vi "Move to point.vi"(11 "Point":T2) -> ()   [LabVIEW 2011]
uses:
  point.ctl
  <vilib>/addons/control/pid/pid.llb/PID (DBL).vi
  <vilib>/addons/control/pid/NI_PID_pid.lvlib
panel:
  in  "Y axix PID gains 2":T1={"proportional gain (Kc)"=0.5, "integral time (Ti, min)"=0.1, "derivative time (Td, min)"=0.0}
  in  "X axis PID gains":T1={"proportional gain (Kc)"=2.0, "integral time (Ti, min)"=0.01, "derivative time (Td, min)"=0.0}
  in  "Y scale":dbl
  in  "X scale":dbl
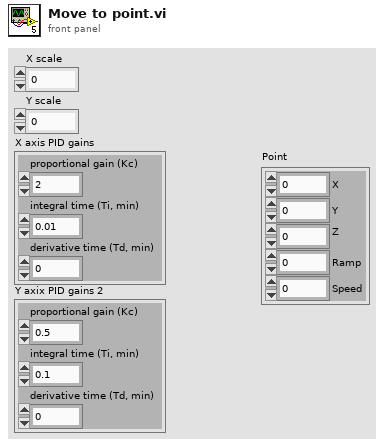
[diagram p1: front panel]
types:
  T1 = cluster{"proportional gain (Kc)":dbl, "integral time (Ti, min)":dbl, "derivative time (Td, min)":dbl}
  T2 = typedef "point.ctl" = cluster{"X":dbl, "Y":dbl, "Z":dbl, "Ramp":dbl, "Speed":dbl}
  T3 = typedef "WPI_EncoderDevRef.ctl" = cluster{"DevStatus":errorcluster, "EncoderIndex":T4, "CounterIndex":T5, "DistancePerCount":dbl, "Decoding Type":T6}
  T4 = typedef "FPGA_EncoderIdx.ctl" = enum8{"Enc 0", "Enc 1", "Enc 2", "Enc 3", "Invalid"}
  T5 = typedef "FPGA_CounterCtrSystemIndex.ctl" = enum8{"Ctr 0", "Ctr 1", "Ctr 2", "Ctr 3", "Ctr 4", "Ctr 5", "Ctr 6", "Ctr 7", "Invalid"}
  T6 = typedef "WPI_EncoderType.ctl" = enum16{"1x", "2x", "4x"}
  T7 = typedef "WPI_MotorControlDeviceRef.ctl" = cluster{"DeviceStatus":errorcluster, "Type":enum16{"PWM", "CAN"}, "PWM":cluster{"Digital Module":T8, "PWM Channel":T9, "DeadBand":T10}, "CAN":cluster{"Device Number":u8, "Control Mode":T11, "Semaphore":T12, "Max Vout":dbl}, "Invert":bool, "TransformRef":T13, "InvTransformRef":T13}
  T8 = typedef "FPGA_TypedefDigitalModule.ctl" = enum16{"Digital Module 1", "Digital Module 2"}
  T9 = typedef "FPGA_DIOPWMChannel.ctl" = enum8{"PWM 1", "PWM 2", "PWM 3", "PWM 4", "PWM 5", "PWM 6", "PWM 7", "PWM 8", "PWM 9", "PWM 10", "Invalid"}
  T10 = typedef "WPI_PWMDeadband.ctl" = cluster{"Name":string, "maxPositivePwm":i32, "minPositivePwm":i32, "centerPwm":i32, "maxNegativePwm":i32, "minNegativePwm":i32, "angularRange":u16}
  T11 = typedef "WPI_CANJaguar_ControlMode.ctl" = enum8{"Percent VBus", "Current", "Speed", "Position", "Voltage"}
  T12 = typedef "Semaphore RefNum" = refnum<k1>
  T13 = typedef "WPI_PWMTransform_ConPane.ctl" = refnum<vi>
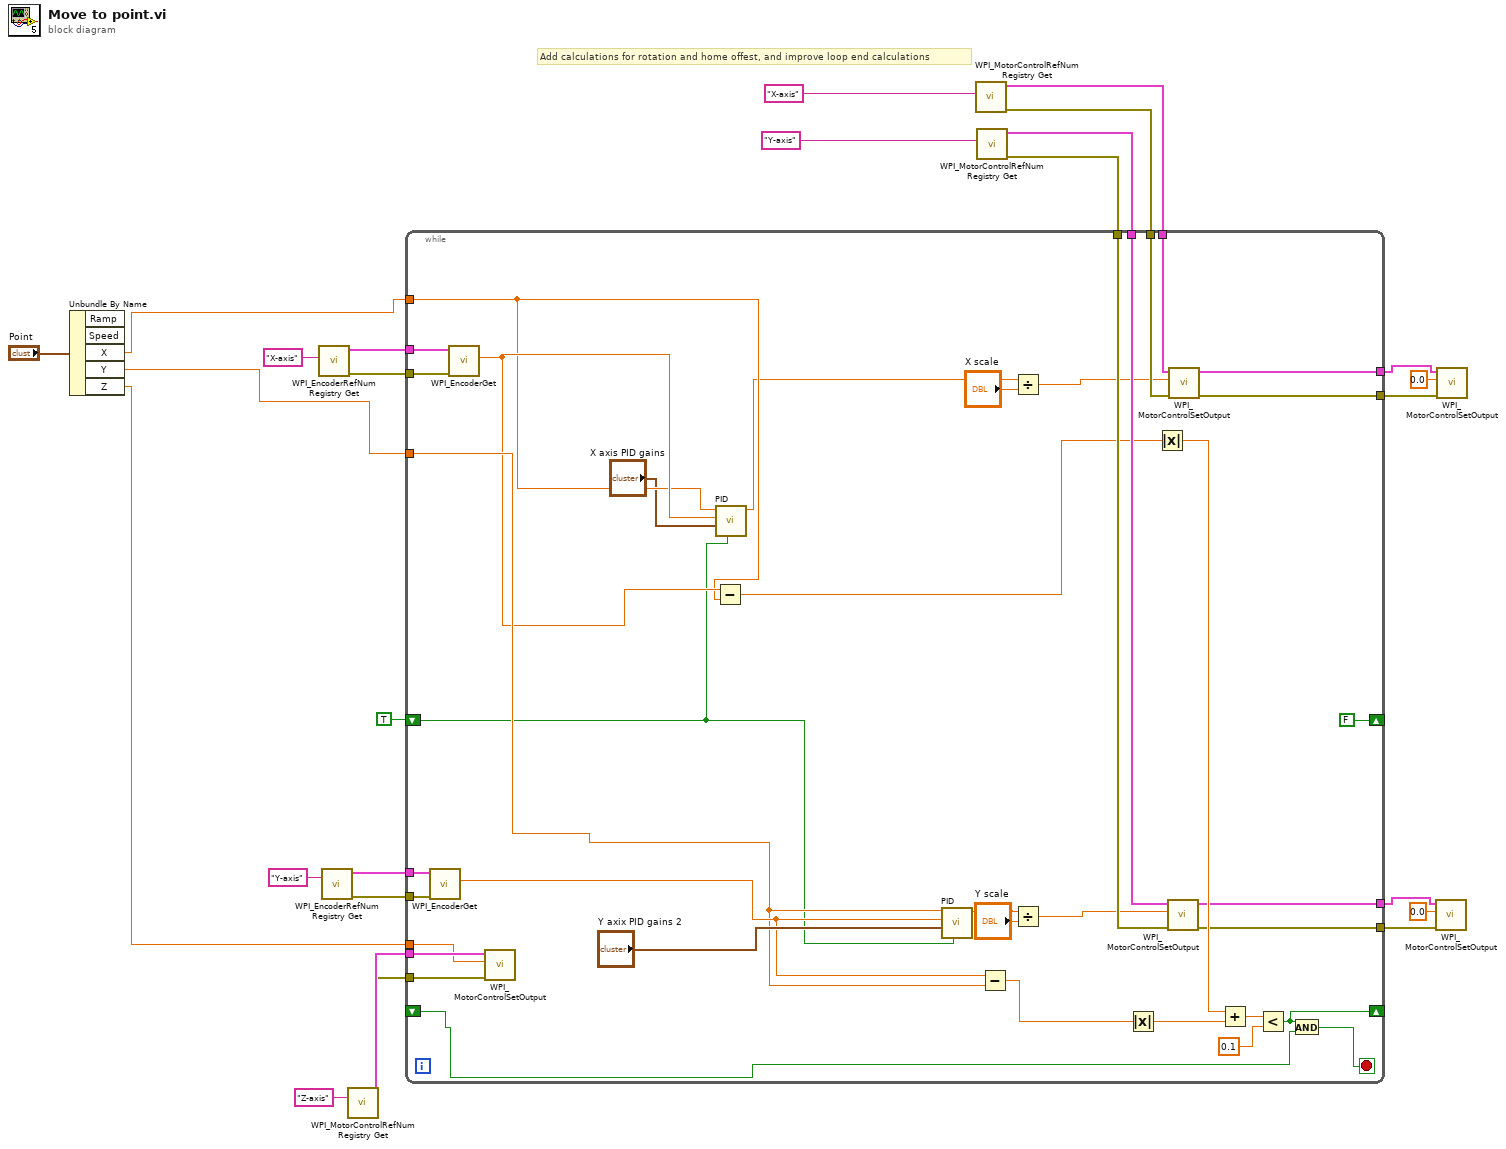
[diagram p0: block diagram]
diagram:
  # "Add calculations for rotation and home offest, and improve loop end calculations"
  n1 = Unbundle By Name("Point") -> ("X"=w8:dbl, "Y"=w9:dbl, "Z"=w10:dbl)  [unwired: 2 out]
  n2 = call <vilib>:"WPI_EncoderRefNum Registry Get.vi"("refnum name"="X-axis") -> ("error out"=w23:errorcluster, "EncoderDevRef"=w22:T3)  [unwired: 9 in]
  n3 = call <vilib>:"WPI_EncoderRefNum Registry Get.vi"("refnum name"="Y-axis") -> ("error out"=w20:errorcluster, "EncoderDevRef"=w21:T3)  [unwired: 9 in]
  n4 = call <vilib>:"WPI_MotorControlRefNum Registry Get.vi"("refnum name"="Z-axis") -> ("error out"=w12:errorcluster, "MotorControlDevRef"=w13:T7)  [unwired: 9 in]
  n5 = call <vilib>:"WPI_MotorControlRefNum Registry Get.vi"("refnum name"="X-axis") -> ("error out"=w17:errorcluster, "MotorControlDevRef"=w18:T7)  [unwired: 9 in]
  n6 = call <vilib>:"WPI_MotorControlRefNum Registry Get.vi"("refnum name"="Y-axis") -> ("error out"=w14:errorcluster, "MotorControlDevRef"=w15:T7)  [unwired: 9 in]
  n7 = while {
    tunnel: w8 -> [w34]
    tunnel: w23 -> [w64]
    tunnel: w22 -> [w63]
    tunnel: w9 -> [w43]
    tunnel: w21 -> [w61]
    tunnel: w20 -> [w60]
    shift-right: [w55] -> _
    shift-left: _ -> [w36]
    tunnel: w18 -> [w54]
    tunnel: w17 -> [w45]
    tunnel: w15 -> [w53]
    tunnel: w14 -> [w52]
    tunnel: w13 -> [w51]
    tunnel: w12 -> [w50]
    tunnel: w10 -> [w44]
    tunnel: [w40] -> w7
    tunnel: [w39] -> w6
    tunnel: [w38] -> w5
    tunnel: [w37] -> w4
    shift-right: [FALSE] -> _
    shift-left: TRUE -> [w28]
    stop <- w31 stop-if-true
    n8 = call <vilib>:"WPI_EncoderGet.vi"("error in (no error)"=w60, "EncoderDevRef"=w61) -> ("Distance"=w46:dbl)  [unwired: 4 in, 5 out]
    n9 = call <vilib>:"WPI_EncoderGet.vi"("error in (no error)"=w64, "EncoderDevRef"=w63) -> ("Distance"=w35:dbl)  [unwired: 4 in, 5 out]
    n10 = call <vilib>:"WPI_MotorControlSetOutput.vi"("error in (no error)"=w50, "Output"=w44, "MotorControlDevRef"=w51) -> ()  [unwired: 7 in, 2 out]
    n11 = Subtract(x=w35, y=w34) -> (x-y=w48:dbl)
    n12 = call-poly <vilib>:"PID.vi"("reinitialize? (F)"=w28, "PID gains"="X axis PID gains", "process variable"=w35, "setpoint"=w34) -> ("output"=w32:dbl)  [unwired: 6 in, 1 out]
    n13 = call-poly <vilib>:"PID.vi"("reinitialize? (F)"=w28, "PID gains"="Y axix PID gains 2", "process variable"=w46, "setpoint"=w43) -> ("output"=w59:dbl)  [unwired: 6 in, 1 out]
    n14 = Subtract(x=w46, y=w43) -> (x-y=w58:dbl)
    n15 = Divide(x=w32, y="X scale") -> (x/y=w42:dbl)
    n16 = Divide(x=w59, y="Y scale") -> (x/y=w41:dbl)
    n17 = Absolute Value(x=w58) -> (abs(x)=w49:dbl)
    n18 = Absolute Value(x=w48) -> (abs(x)=w47:dbl)
    n19 = call <vilib>:"WPI_MotorControlSetOutput.vi"("error in (no error)"=w52, "Output"=w41, "MotorControlDevRef"=w53) -> ("error out"=w38:errorcluster, "MotorControlDevRef"=w39:T7)  [unwired: 7 in]
    n20 = call <vilib>:"WPI_MotorControlSetOutput.vi"("error in (no error)"=w45, "Output"=w42, "MotorControlDevRef"=w54) -> ("error out"=w37:errorcluster, "MotorControlDevRef"=w40:T7)  [unwired: 7 in]
    n21 = Add(x=w47, y=w49) -> (x+y=w57:dbl)
    n22 = Less?(x=w57, y=0.1) -> (x < y?=w55:bool)
    n23 = And(x=w55, y=w36) -> (x .and. y?=w31:bool)
  }
  n24 = call <vilib>:"WPI_MotorControlSetOutput.vi"("error in (no error)"=w5, "Output"=0.0, "MotorControlDevRef"=w6) -> ()  [unwired: 7 in, 2 out]
  n25 = call <vilib>:"WPI_MotorControlSetOutput.vi"("error in (no error)"=w4, "Output"=0.0, "MotorControlDevRef"=w7) -> ()  [unwired: 7 in, 2 out]
